vi "Draw Help.vi"(10 "Display Help":bool, 11 "Screen in":picture) -> (3 "Screen out":picture)   [LabVIEW 2020, in "Example 1.lvlib"]
uses:
  Example 1.lvlib
  9f43915e-2be4-4177-985d-f5d8817b1a37.vi
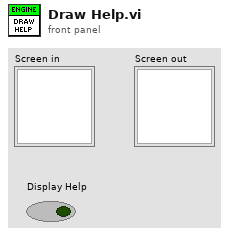
[diagram p1: front panel]
types:
  T1 = enum16{"User-specified Font", "Application Font", "System Font", "Dialog Font"}
  T2 = cluster{"Font Name:":string, "Size":i16, "Strikeout?":bool, "Italic?":bool, "Underline?":bool, "Outline?":bool, "Shadow?":bool, "Bold?":bool}
  T3 = cluster{"left":i16, "top":i16, "right":i16, "bottom":i16}
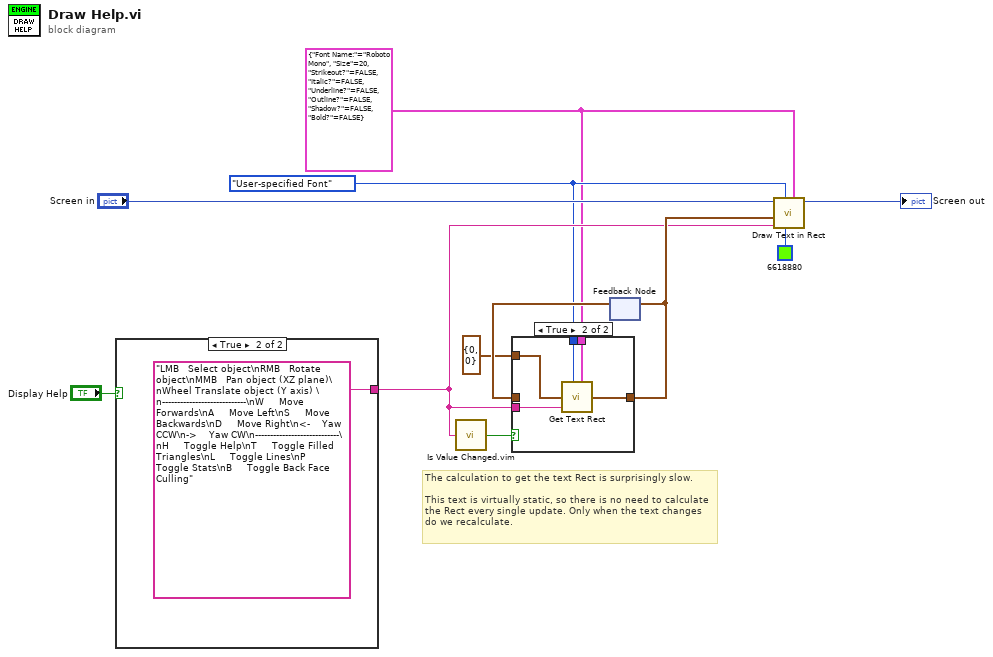
[diagram p0: block diagram]
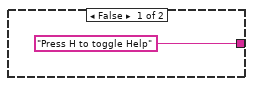
[diagram p3: hidden frame]
diagram:
  w3 = T1."User-specified Font" ("desired font(Application)")
  w2 = T2 {"Font Name:"="Roboto Mono", "Size"=20, "Strikeout?"=FALSE, "Italic?"=FALSE, "Underline?"=FALSE, "Outline?"=FALSE, "Shadow?"=FALSE, "Bold?"=FALSE} ("[user-specified font]")
  # "The calculation to get the text Rect is surprisingly slow.\n\nThis text is virtually static, so there is no need to calculate the Rect every single update. Only when the text changes do we recalculate."
  n1 = case shown="True" "Display Help" {
    tunnel: ["Press H to toggle Help" ("text") "LMB   Select object\nRMB   Rotate object\nMMB   Pan object (XZ plane)\nWheel Translate object (Y axis) \n----------------------------\nW     Move Forwards\nA     Move Left\nS     Move Backwards\nD     Move Right\n<-    Yaw CCW\n->    Yaw CW\n----------------------------\nH     Toggle Help\nT     Toggle Filled Triangles\nL     Toggle Lines\nP     Toggle Stats\nB     Toggle Back Face Culling" ("text")] -> w4
    frame False {
    }
    frame True {
    }
  }
  n2 = call "Is Value Changed.vim"("value"=w4) -> ("changed or first call?"=w7:bool)
  n3 = feedback #1() -> (w6:T3)  [unwired: 1 in]
  n4 = case shown="True" w7 {
    tunnel: [w14 w19] -> w5
    tunnel: w6 -> [w14 _]
    tunnel: cluster{"x":i16, "y":i16} {"x"=0, "y"=0} ("origin") -> [_ w18]
    tunnel: w3 -> [_ w17]
    tunnel: w2 -> [_ w16]
    tunnel: w4 -> [_ w15]
    frame False {
    }
    frame True {
      n5 = call <vilib>:"Get Text Rect.vi"("desired font(Application)"=w17, "origin(0,0)"=w18, "text"=w15, "[user-specified font]"=w16) -> ("rect"=w19:T3)  [unwired: 5 in]
    }
  }
  n6 = feedback-in #1(w5) -> ()
  n7 = call <vilib>:"Draw Text in Rect.vi"("[user-specified font]"=w2, "text color(black)"=u32 6618880, "desired font(Application)"=w3, "text"=w4, "rect"=w5, "picture"="Screen in") -> ("new picture"=→"Screen out":picture)  [unwired: 5 in]
